vi "project.vi"() -> ()   [LabVIEW 2021]
uses:
  <vilib>/LabVIEW Interface for Arduino/Type Defs/Board Type.ctl
  <vilib>/LabVIEW Interface for Arduino/Type Defs/Connection Type.ctl
  <vilib>/LabVIEW Interface for Arduino/Type Defs/Pin Mode.ctl
  <vilib>/LabVIEW Interface for Arduino/LabVIEW Interface for Arduino.lvlib
panel:
  in  "stop":bool
  out "Boolean":bool
  out "Waveform Chart":dbl(graph)
  out "Analog signal":dbl(knob) scale=0.0..500.0
  in  "VISA resource":refnum<visa-resource-name>
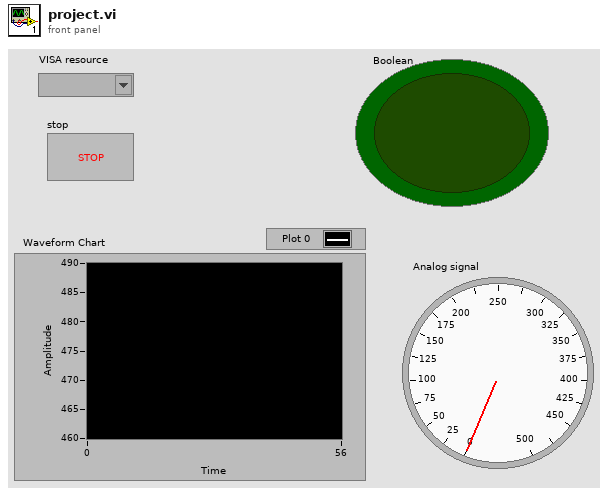
[diagram p1: front panel]
types:
  T1 = typedef "LabVIEW Interface for Arduino.lvlib/Connection Type.ctl" = enum8{"USB / Serial", "XBEE", "BlueSmirf (Bluetooth)"}
  T2 = typedef "LabVIEW Interface for Arduino.lvlib/Board Type.ctl" = enum16{"Uno", "Dimuelanove w/Atmega 328", "Mega 2560"}
  T3 = typedef "LabVIEW Interface for Arduino.lvlib/Arduino Resource.ctl" = cluster{"VISA resource":refnum<visa-resource-name>, "Board Type":T2, "Connection Type":enum8{"USB / Serial"}, "Bytes Per Packet (15)":u8}
  T4 = typedef "LabVIEW Interface for Arduino.lvlib/Pin Mode.ctl" = enum8{"Input", "Output"}
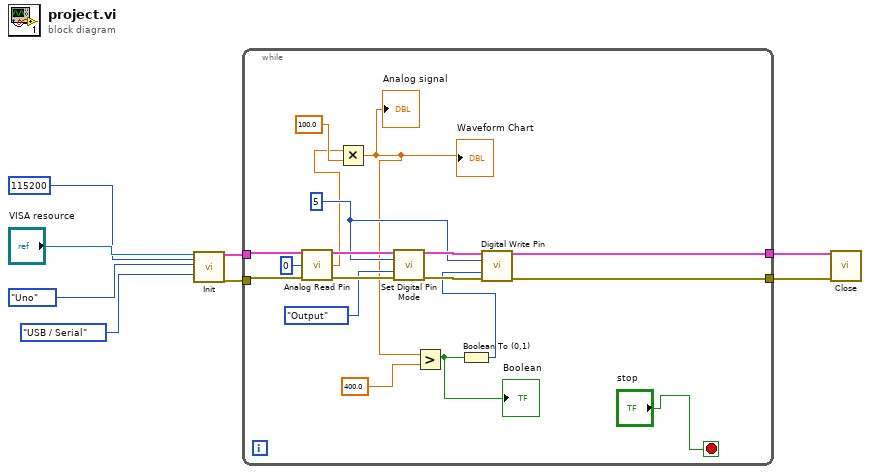
[diagram p0: block diagram]
diagram:
  n1 = call <vilib>:"Init.vi"("VISA resource"="VISA resource", "Baud Rate (115200)"=u32 115200, "Board Type (Uno)"=Board_Type."Uno", "Connection Type (USB/Serial)"=Connection_Type."USB / Serial") -> ("Arduino Resource"=w4:T3, "error out"=w3:errorcluster)  [unwired: 14 in]
  n2 = while {
    tunnel: w4 -> [w26]
    tunnel: w3 -> [w25]
    tunnel: [w22] -> w2
    tunnel: [w21] -> w1
    stop <- "stop" stop-if-true
    w16 = u8 5 ("Digital I/O Pin")
    n3 = call <vilib>:"Analog Read Pin.vi"("Arduino Resource"=w26, "Analog Input Pin (0)"=u8 0, "error in"=w25) -> ("Arduino Resource"=w24:T3, "Voltage"=w14:dbl, "error out"=w19:errorcluster)  [unwired: 10 in]
    n4 = Multiply(x=w14, y=100.0) -> (x*y=w9:dbl)
    "Analog signal" <- w9
    "Waveform Chart" <- w9
    n5 = call <vilib>:"Set Digital Pin Mode.vi"("Arduino Resource"=w24, "Digital I/O Pin"=w16, "Pin Mode (Input)"=Pin_Mode."Output", "error in"=w19) -> ("Arduino Resource"=w23:T3, "error out"=w20:errorcluster)  [unwired: 10 in]
    n6 = Greater?(x=w9, y=400.0) -> (0:w11:bool)
    "Boolean" <- w11
    n7 = Boolean To (0,1)(Boolean=w11) -> (0, 1=w12:i16)
    n8 = call <vilib>:"Digital Write Pin.vi"("Arduino Resource"=w23, "Digital I/O Pin (0)"=w16, "Value (0)"=w12, "error in"=w20) -> ("Arduino Resource"=w22:T3, "error out"=w21:errorcluster)  [unwired: 10 in]
  }
  n9 = call <vilib>:"Close.vi"("Arduino Resource"=w2, "error in"=w1) -> ()  [unwired: 13 in, 1 out]
